vi "Lookup Config.vi"(7 "Context (Root)":refnum<class "Config Element.lvclass">, 8 "error in (no error)":errorcluster, 10 "Lookup":refnum<class "Config Lookup.lvclass">, 11 "Config Manager in":refnum<class "Config Manager.lvclass">) -> (0 "error out":errorcluster, 2 "Matches":refnum<class "Config Element.lvclass">[](array[class]), 3 "Config Manager out":refnum<class "Config Manager.lvclass">)   [LabVIEW 2020, in "CDM-Config.lvlib" / "Config Manager.lvclass"]
uses:
  Config Manager.lvclass
  Config Lookup/Config Lookup.lvclass
  Config Element/Config Element.lvclass
  Config Element/Config Element.lvclass/Config Element.ctl
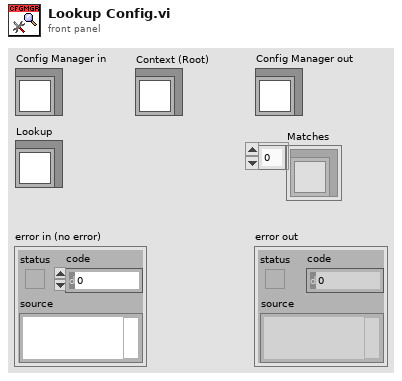
[diagram p1: front panel]
types:
  T1 = typedef "CDM-Config.lvlib/Meta Data.ctl" = cluster{"Name":string, "Value":string}
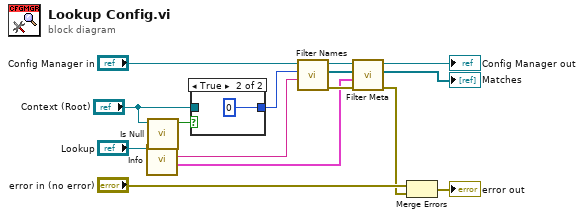
[diagram p0: block diagram]
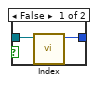
[diagram p2: hidden frame]
diagram:
  n1 = call "Info.vi"("Config Lookup in"="Lookup") -> ("Meta"=w5:T1[], "Name"=w8:string)  [unwired: 9 in]
  n2 = call "Is Null.vi"("Config Element in"="Context (Root)") -> ("Null"=w11:bool)  [unwired: 10 in]
  n3 = case shown="True" w11 {
    tunnel: "Context (Root)" -> [w17 _]
    tunnel: [w16 0 ("Index")] -> w9
    frame False {
      n4 = call "Index.vi"("Config Element in"=w17) -> ("Index"=w16:i32)  [unwired: 9 in, 1 out]
    }
    frame True {
    }
  }
  n5 = call "Filter Names.vi"("Name"=w8, "Root Index"=w9, "Config Manager in"="Config Manager in") -> ("error out"=w15:errorcluster, "Elements"=w6:refnum<class "Config Element.lvclass">[], "Config Manager out"=w7:refnum<class "Config Manager.lvclass">)  [unwired: 6 in]
  n6 = call "Filter Meta.vi"("error in (no error)"=w15, "Meta"=w5, "Elements"=w6, "Config Manager in"=w7) -> ("error out"=w1:errorcluster, "Matches"=→"Matches":refnum<class "Config Element.lvclass">[], "Config Manager out"=→"Config Manager out":refnum<class "Config Manager.lvclass">)  [unwired: 5 in]
  n7 = Merge Errors("error in (no error)", w1) -> (→"error out":errorcluster)
